vi "Setup Framework.vi"() -> (0 "error out":errorcluster, 2 "Message Queues":T1, 3 "Events":T2)   [LabVIEW 2023, in "HAF.lvlib"]
doc: "Initialises the Framework for operation by creating the Events and Message Queues that are required by the Framework and, most likely, the Application.\n\nThis should always be called before the framework is tasked with doing anything."
uses:
  HAF.lvlib
  All Events.ctl
  Stop Event.ctl
  Event Data.ctl
  Pause Event.ctl
  Resume Event.ctl
  Done Event.ctl
  Injection Event.ctl
  All Message Queues.ctl
  Message.ctl
  Global Resources.vi
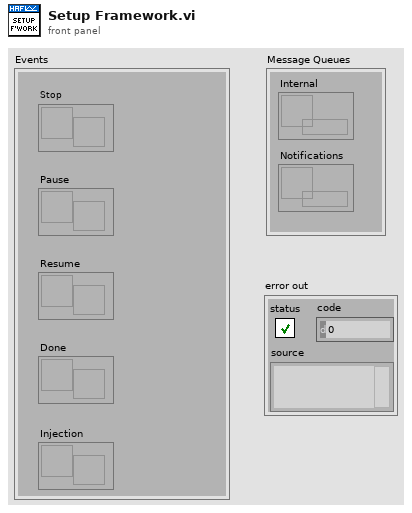
[diagram p1: front panel]
types:
  T1 = typedef "HAF.lvlib/All Message Queues.ctl" = cluster{"Internal":refnum<queue>, "Notifications":refnum<queue>}
  T2 = typedef "HAF.lvlib/All Events.ctl" = cluster{"Stop":T3, "Pause":T4, "Resume":T5, "Done":T6, "Injection":T7}
  T3 = typedef "HAF.lvlib/Stop Event.ctl" = refnum<user-event>
  T4 = typedef "HAF.lvlib/Pause Event.ctl" = refnum<user-event>
  T5 = typedef "HAF.lvlib/Resume Event.ctl" = refnum<user-event>
  T6 = typedef "HAF.lvlib/Done Event.ctl" = refnum<user-event>
  T7 = typedef "HAF.lvlib/Injection Event.ctl" = refnum<user-event>
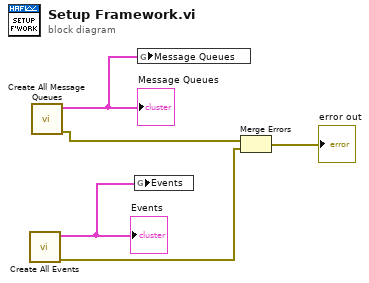
[diagram p0: block diagram]
diagram:
  n1 = call "Create All Events.vi"() -> ("error out"=w4:errorcluster, "Events"=w1:T2)  [unwired: 10 in]
  "Events" <- w1
  n2 = call "Create All Message Queues.vi"() -> ("error out"=w5:errorcluster, "Message Queues"=w2:T1)  [unwired: 10 in]
  "Message Queues" <- w2
  n3 = global write "Global Resources.vi" "Events"(w1) -> ()
  n4 = global write "Global Resources.vi" "Message Queues"(w2) -> ()
  n5 = Merge Errors(w5, w4) -> (→"error out":errorcluster)
